vi "PH_gentec_Powermeter.set wanted Sets to GUI.vi"(0 "i ref in":refnum<vi>, 5 "error in":errorcluster) -> (14 "i ref out":refnum<vi>, 19 "error out":errorcluster)   [LabVIEW 2014, in "PH_gentec_Powermeter.lvlib"]
doc: "This VI indicates the wanted Settings at the GUI element."
uses:
  PH_gentec_Powermeter.lvlib
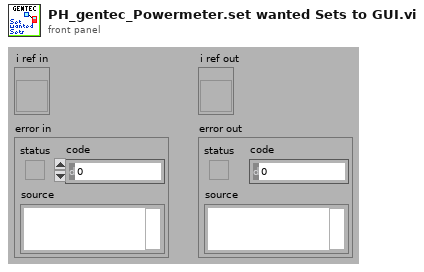
[diagram p1: front panel]
types:
  T1 = typedef "PH_gentec_Powermeter.lvlib/PH_gentec_Powermeter.i attribute.ctl" = cluster{"GUI References":cluster{"delete":refnum<vi>, "start stop Statistics":refnum<vi>, "Statistic Data":refnum<vi>, "Configuration Values":refnum<vi>, "Set Zero":refnum<vi>, "Data Sampling Settings":refnum<vi>, "Wanted Sets":refnum<vi>, "Current Sets":refnum<vi>}, "Start Stop Statistics":bool, "Wanted Sets":T2, "Current Sets":T2}
  T2 = typedef "PH_gentec_Powermeter.lvlib/PH_gentec_Powermeter.Sets.ctl" = cluster{"Data Sampling Settings":T3, "Set Zero":bool}
  T3 = typedef "gentec-SOLO-PE - Driver.lvlib/gentec-SOLO-PE.Data Sampling Settings.ctl" = cluster{"Sample Rate":u32, "Sample Rate Unit":u32, "Sample Period":u32, "Sample Period Unit":u32, "Total Duration":u32, "Total Duration Unit":u32, "Time Stamp":u32}
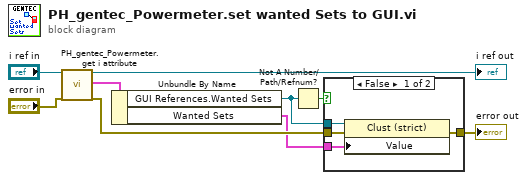
[diagram p0: block diagram]
diagram:
  n1 = call "PH_gentec_Powermeter.get i attribute.vi"("i ref in"="i ref in", "error in (no error)"="error in") -> ("i ref out"=→"i ref out":refnum<vi>, "i attribute"=w8:T1, "error out"=w6:errorcluster)  [unwired: 15 in]
  n2 = Unbundle By Name(w8) -> ("GUI References.Wanted Sets"=w5:refnum<vi>, "Wanted Sets"=w1:T2)
  n3 = Not A Number/Path/Refnum?(number/path/refnum=w5) -> (NaN/Path/Refnum?=w2:bool)
  n4 = case shown="False" w2 {
    tunnel: [w12 w14] -> w9
    tunnel: w5 -> [w11 _]
    tunnel: w6 -> [w13 w14]
    tunnel: w1 -> [w10 _]
    frame False {
      n5 = property class="Clust (strict)"(reference=w11, error in=w13, "Value"=w10) -> (error out=w12:errorcluster)  [unwired: 1 out]
    }
    frame True {
    }
  }
  "error out" <- w9
